vi "Handle Value Change - Add to Virtual Folder.vi"(8 "Error In":errorcluster, 10 "New Value":bool, 11 "Module Data In":T1) -> (0 "Error Out":errorcluster)   [LabVIEW 2022 SP3]
doc: "This VI handles the Value Change event on the \"Add To Virtual Folder?\" checkbox.\n\nAcronyms\nATP = \"Add To Project?\" checkbox\nATO = \"Add To Owner?\" checkbox\nATVF = \"Add To Virtual Folder?\" checkbox"
uses:
  Module Data.ctl
  GUI Object Refs (cluster).ctl
  Initial State (enum).ctl
  Input Conditions (cluster).ctl
  DFS Output (cluster).ctl
panel:
  # "Development\nControls or indicators that are useful for development or testing, but which are not outputs of the VI."
  # "Input\nInputs to the VI"
  # "Output\nOutputs of the VI"
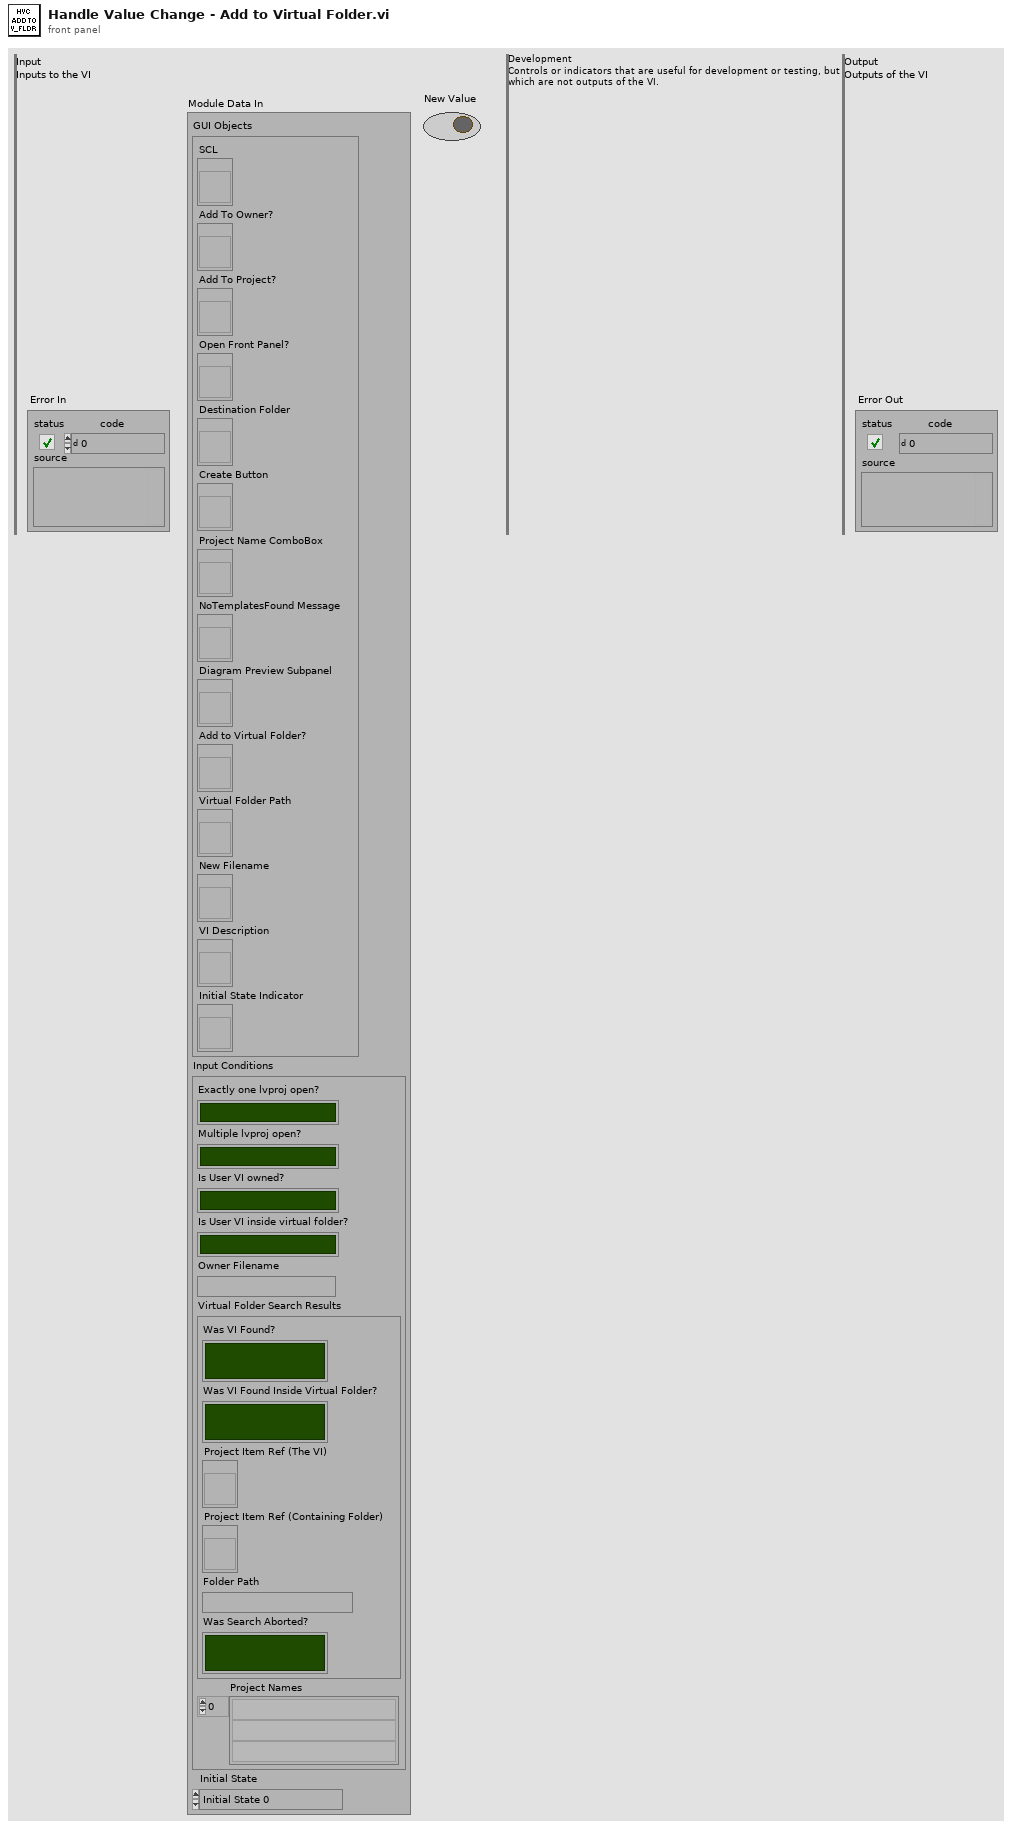
[diagram p1: front panel]
types:
  T1 = typedef "Module Data.ctl" = cluster{"GUI Objects":T2, "Input Conditions":T3, "Initial State":T5}
  T2 = typedef "GUI Object Refs (cluster).ctl" = cluster{"SCL":refnum<vi>, "Add To Owner?":refnum<vi>, "Add To Project?":refnum<vi>, "Open Front Panel?":refnum<vi>, "Destination Folder":refnum<vi>, "Create Button":refnum<vi>, "Project Name ComboBox":refnum<vi>, "NoTemplatesFound Message":refnum<vi>, "Diagram Preview Subpanel":refnum<vi>, "Add to Virtual Folder?":refnum<vi>, "Virtual Folder Path":refnum<vi>, "New Filename":refnum<vi>, "VI Description":refnum<vi>, "Initial State Indicator":refnum<vi>}
  T3 = typedef "Input Conditions (cluster).ctl" = cluster{"Exactly one lvproj open?":bool, "Multiple lvproj open?":bool, "Is User VI owned?":bool, "Is User VI inside virtual folder?":bool, "Owner Filename":string, "Virtual Folder Search Results":T4, "Project Names":string[]}
  T4 = typedef "DFS Output (cluster).ctl" = cluster{"Was VI Found?":bool, "Was VI Found Inside Virtual Folder?":bool, "Project Item Ref (The VI)":refnum<vi>, "Project Item Ref (Containing Folder)":refnum<vi>, "Folder Path":string, "Was Search Aborted?":bool}
  T5 = typedef "Initial State (enum).ctl" = enum16{"Initial State 0", "Initial State 1", "Initial State 2", "Initial State 3", "Initial State 4", "Initial State 5", "Initial State 6", "Initial State 7", "Initial State 8", "Initial State 9", "Initial State 10", "Initial State 11", "Initial State 12", "Initial State 13", "Initial State 14", "Initial State 15"}
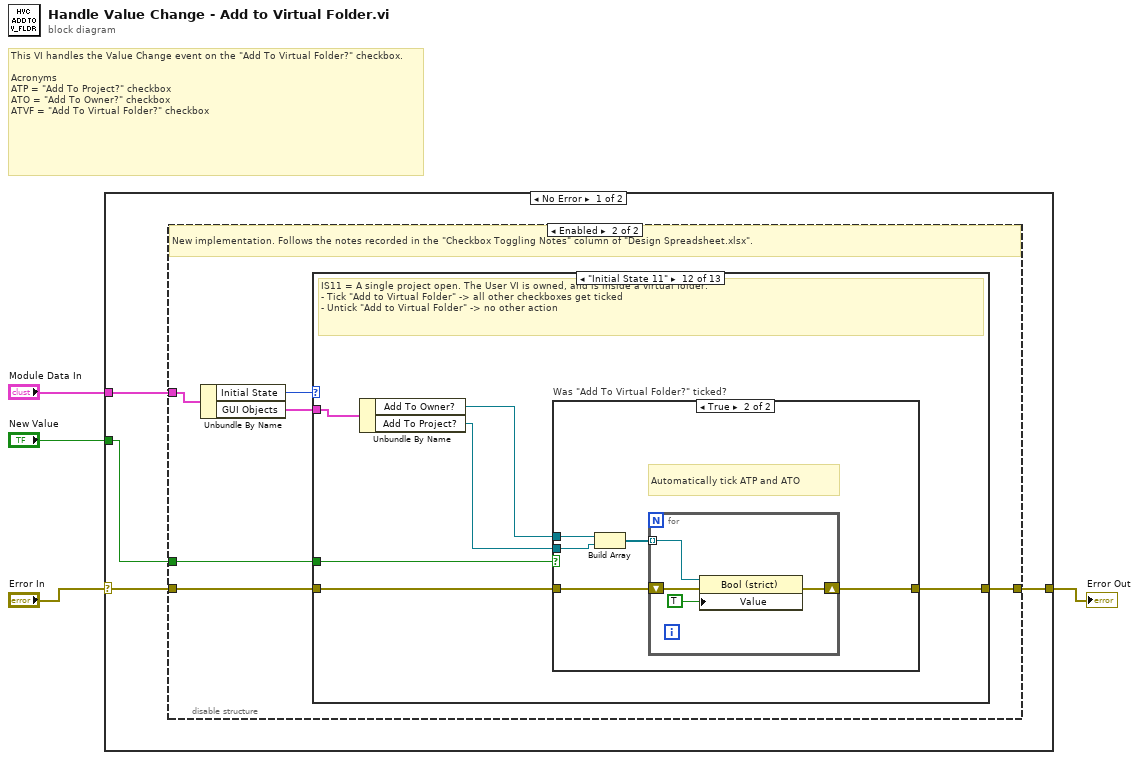
[diagram p0: block diagram]
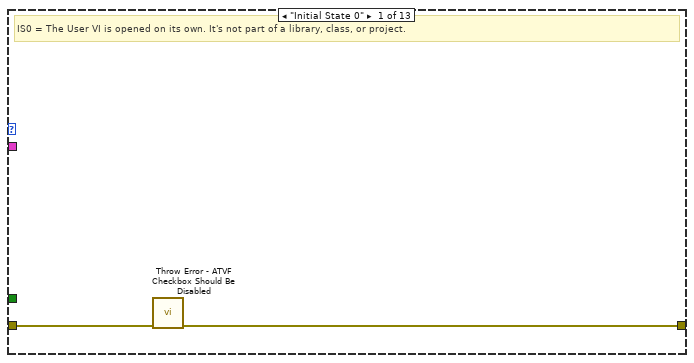
[diagram p3: hidden frame]
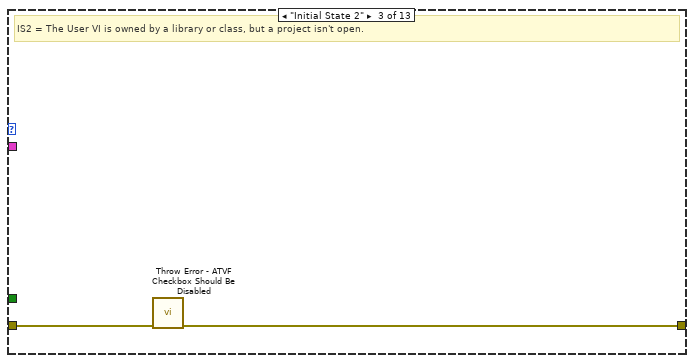
[diagram p5: hidden frame]
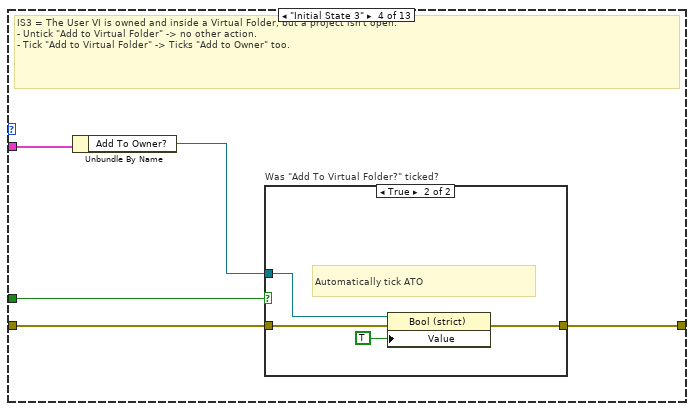
[diagram p6: hidden frame]
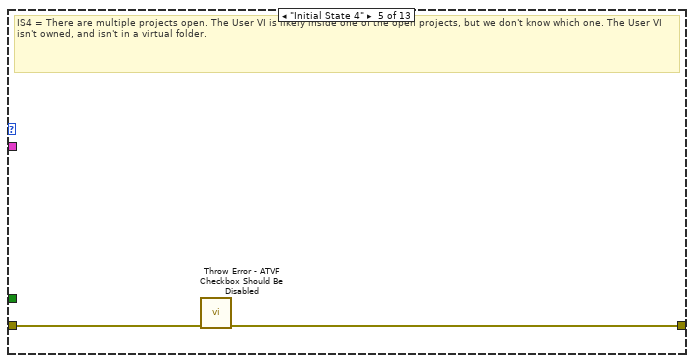
[diagram p8: hidden frame]
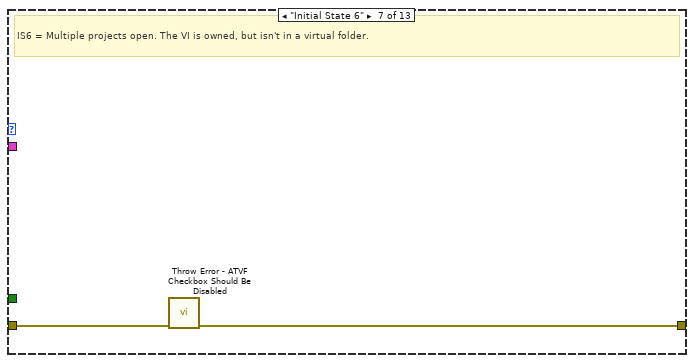
[diagram p10: hidden frame]
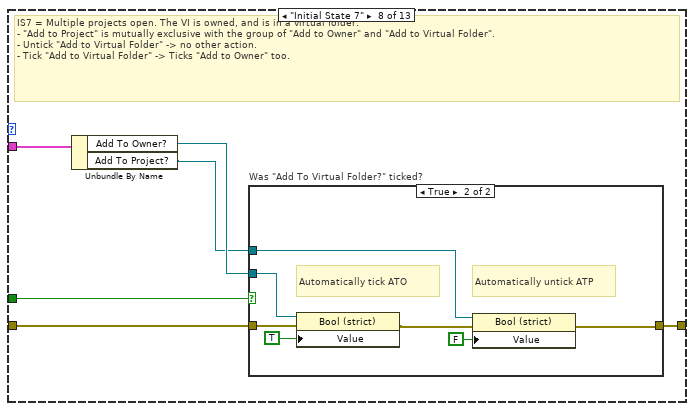
[diagram p11: hidden frame]
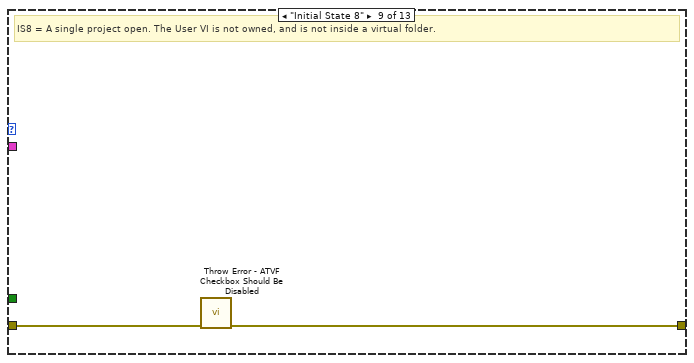
[diagram p13: hidden frame]
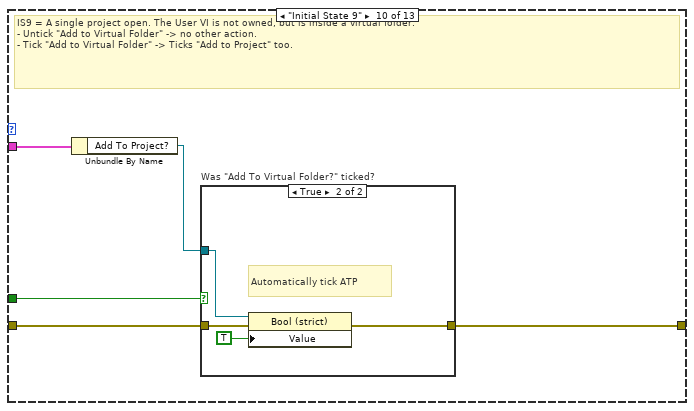
[diagram p14: hidden frame]
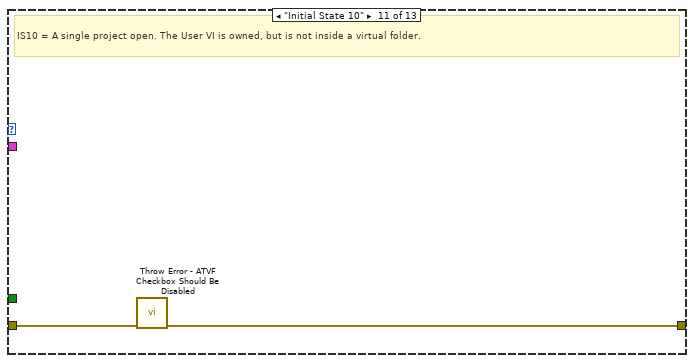
[diagram p16: hidden frame]
diagram:
  # "This VI handles the Value Change event on the \"Add To Virtual Folder?\" checkbox.\n\nAcronyms\nATP = \"Add To Project?\" checkbox\nATO = \"Add To Owner?\" checkbox\nATVF = \"Add To Virtual Folder?\" checkbox"
  n1 = case shown="No Error" "Error In" {
    selector: "Error In" -> [w8 w81]
    tunnel: [w7 w81] -> w3
    tunnel: "Module Data In" -> [w6 _]
    tunnel: "New Value" -> [w5 _]
    frame No Error {
      n2 = disable-structure shown="Enabled" {
        disable-tunnel: w8 -> [w9 w15]
        disable-tunnel: [w9 w13] -> w7
        disable-tunnel: w6 -> [_ w14]
        disable-tunnel: w5 -> [_ w11]
        frame Disabled {
          # "Old implementation. Before 11 Dec 2022."
        }
        frame Enabled {
          # "New implementation. Follows the notes recorded in the \"Checkbox Toggling Notes\" column of \"Design Spreadsheet.xlsx\"."
          n3 = Unbundle By Name(w14) -> ("Initial State"=w12:T5, "GUI Objects"=w10:T2)
          n4 = case shown="\"Initial State 11\"" w12 {
            tunnel: w15 -> [w17 w18 w20 w24 w32 w33 w35 w40 w51 w56 w63 w68 w80]
            tunnel: [w16 w18 w19 w23 w31 w33 w34 w39 w50 w55 w62 w65 w80] -> w13
            tunnel: w11 -> [_ _ _ w22 _ _ _ w38 _ w54 _ w67 _]
            tunnel: w10 -> [_ _ _ w21 _ _ _ w37 _ w53 _ w66 _]
            frame "Initial State 0" {
              # "IS0 = The User VI is opened on its own. It's not part of a library, class, or project."
              n5 = call "Throw Error - ATVF Checkbox Should Be Disabled.vi"("error in"=w17) -> ("error out"=w16:errorcluster)  [unwired: 10 in]
            }
            frame "Initial State 1" {
              # "Impossible Initial State. Expected to never occur."
            }
            frame "Initial State 2" {
              # "IS2 = The User VI is owned by a library or class, but a project isn't open."
              n6 = call "Throw Error - ATVF Checkbox Should Be Disabled.vi"("error in"=w20) -> ("error out"=w19:errorcluster)  [unwired: 10 in]
            }
            frame "Initial State 3" {
              # "IS3 = The User VI is owned and inside a Virtual Folder, but a project isn't open.\n- Untick \"Add to Virtual Folder\" -> no other action.\n- Tick \"Add to Virtual Folder\" -> Ticks \"Add to Owner\" too."
              n7 = Unbundle By Name(w21) -> ("Add To Owner?"=w25:refnum<vi>)
              n8 = case "Was \"Add To Virtual Folder?\" ticked?" shown="True" w22 {
                tunnel: w24 -> [w26 w30]
                tunnel: [w26 w29] -> w23
                tunnel: w25 -> [_ w28]
                frame False {
                  # "Do nothing."
                }
                frame True {
                  # "Automatically tick ATO"
                  n9 = property class="Bool (strict)"(reference=w28, error in=w30, "Value"=TRUE) -> (error out=w29:errorcluster)  [unwired: 1 out]
                }
              }
            }
            frame "Initial State 4" {
              # "IS4 = There are multiple projects open. The User VI is likely inside one of the open projects, but we don't know which one. The User VI isn't owned, and isn't in a virtual folder."
              n10 = call "Throw Error - ATVF Checkbox Should Be Disabled.vi"("error in"=w32) -> ("error out"=w31:errorcluster)  [unwired: 10 in]
            }
            frame "Initial State 5" {
              # "Impossible Initial State. Expected to never occur."
            }
            frame "Initial State 6" {
              # "IS6 = Multiple projects open. The VI is owned, but isn't in a virtual folder."
              n11 = call "Throw Error - ATVF Checkbox Should Be Disabled.vi"("error in"=w35) -> ("error out"=w34:errorcluster)  [unwired: 10 in]
            }
            frame "Initial State 7" {
              # "IS7 = Multiple projects open. The VI is owned, and is in a virtual folder.\n- \"Add to Project\" is mutually exclusive with the group of \"Add to Owner\" and \"Add to Virtual Folder\".\n- Untick \"Add to Virtual Folder\" -> no other action.\n- Tick \"Add to Virtual Folder\" -> Ticks \"Add to Owner\" too."
              n12 = Unbundle By Name(w37) -> ("Add To Owner?"=w41:refnum<vi>, "Add To Project?"=w36:refnum<vi>)
              n13 = case "Was \"Add To Virtual Folder?\" ticked?" shown="True" w38 {
                tunnel: w40 -> [w42 w49]
                tunnel: [w42 w44] -> w39
                tunnel: w41 -> [_ w48]
                tunnel: w36 -> [_ w43]
                frame False {
                  # "Do nothing."
                }
                frame True {
                  # "Automatically untick ATP"
                  # "Automatically tick ATO"
                  n14 = property class="Bool (strict)"(reference=w48, error in=w49, "Value"=TRUE) -> (error out=w45:errorcluster)  [unwired: 1 out]
                  n15 = property class="Bool (strict)"(reference=w43, error in=w45, "Value"=FALSE) -> (error out=w44:errorcluster)  [unwired: 1 out]
                }
              }
            }
            frame "Initial State 8" {
              # "IS8 = A single project open. The User VI is not owned, and is not inside a virtual folder."
              n16 = call "Throw Error - ATVF Checkbox Should Be Disabled.vi"("error in"=w51) -> ("error out"=w50:errorcluster)  [unwired: 10 in]
            }
            frame "Initial State 9" {
              # "IS9 = A single project open. The User VI is not owned, but is inside a virtual folder.\n- Untick \"Add to Virtual Folder\" -> no other action.\n- Tick \"Add to Virtual Folder\" -> Ticks \"Add to Project\" too."
              n17 = Unbundle By Name(w53) -> ("Add To Project?"=w52:refnum<vi>)
              n18 = case "Was \"Add To Virtual Folder?\" ticked?" shown="True" w54 {
                tunnel: w56 -> [w57 w61]
                tunnel: [w57 w59] -> w55
                tunnel: w52 -> [_ w58]
                frame False {
                  # "Do nothing."
                }
                frame True {
                  # "Automatically tick ATP"
                  n19 = property class="Bool (strict)"(reference=w58, error in=w61, "Value"=TRUE) -> (error out=w59:errorcluster)  [unwired: 1 out]
                }
              }
            }
            frame "Initial State 10" {
              # "IS10 = A single project open. The User VI is owned, but is not inside a virtual folder."
              n20 = call "Throw Error - ATVF Checkbox Should Be Disabled.vi"("error in"=w63) -> ("error out"=w62:errorcluster)  [unwired: 10 in]
            }
            frame "Initial State 11" {
              # "IS11 = A single project open. The User VI is owned, and is inside a virtual folder.\n- Tick \"Add to Virtual Folder\" -> all other checkboxes get ticked\n- Untick \"Add to Virtual Folder\" -> no other action"
              n21 = Unbundle By Name(w66) -> ("Add To Owner?"=w69:refnum<vi>, "Add To Project?"=w64:refnum<vi>)
              n22 = case "Was \"Add To Virtual Folder?\" ticked?" shown="True" w67 {
                tunnel: w68 -> [w70 w75]
                tunnel: [w70 w74] -> w65
                tunnel: w69 -> [_ w73]
                tunnel: w64 -> [_ w71]
                frame False {
                  # "Do nothing."
                }
                frame True {
                  # "Automatically tick ATP and ATO"
                  n23 = Build Array(w73, w71) -> (w72:refnum<vi>[])
                  n24 = for {
                    tunnel: w72 -> [w76] mode=indexing
                    shift-right: [w78] -> w74
                    shift-left: w75 -> [w79]
                    n25 = property class="Bool (strict)"(reference=w76, error in=w79, "Value"=TRUE) -> (error out=w78:errorcluster)  [unwired: 1 out]
                  }
                }
              }
            }
            frame "Initial State 12".."Initial State 15" {
              # "Impossible Initial State. Expected to never occur."
            }
          }
        }
      }
    }
    frame Error {
    }
  }
  "Error Out" <- w3
